vi "arm_cmd_to_duty.vi"(9 "arm_down_signal":u8, 10 "arm_up_signal":u8) -> (2 "duty":dbl)   [LabVIEW 2020]
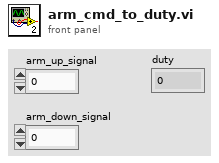
[diagram p1: front panel]
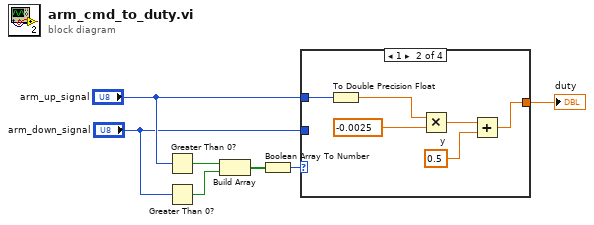
[diagram p0: block diagram]
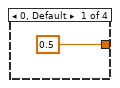
[diagram p2: hidden frame]
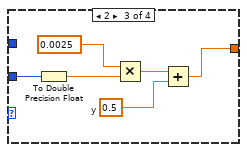
[diagram p3: hidden frame]
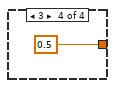
[diagram p4: hidden frame]
diagram:
  n1 = Greater Than 0?(x="arm_up_signal") -> (x > 0?=w7:bool)
  n2 = Greater Than 0?(x="arm_down_signal") -> (x > 0?=w6:bool)
  n3 = Build Array(w7, w6) -> (w5:bool[])
  n4 = Boolean Array To Number(Boolean array=w5) -> (number=w4:u32)
  n5 = case shown="1" w4 {
    tunnel: "arm_up_signal" -> [_ w14 _ _]
    tunnel: "arm_down_signal" -> [_ _ w18 _]
    tunnel: [0.5 w9 w19 0.5] -> w1
    frame 0, Default {
    }
    frame 1 {
      w10 = 0.5  # y
      n6 = To Double Precision Float(number=w14) -> (double precision float=w12:dbl)
      n7 = Multiply(x=w12, y=-0.0025) -> (x*y=w11:dbl)
      n8 = Add(x=w11, y=w10) -> (x+y=w9:dbl)
    }
    frame 2 {
      w20 = 0.5  # y
      n9 = To Double Precision Float(number=w18) -> (double precision float=w16:dbl)
      n10 = Multiply(x=0.0025, y=w16) -> (x*y=w15:dbl)
      n11 = Add(x=w15, y=w20) -> (x+y=w19:dbl)
    }
    frame 3 {
    }
  }
  "duty" <- w1
